vi "PadString.vi"(9 "size":i32=8, 11 "data":string) -> (3 "String":string)   [LabVIEW 2022 SP3]
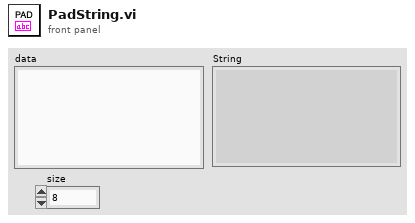
[diagram p1: front panel]
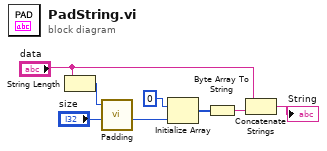
[diagram p0: block diagram]
diagram:
  n1 = String Length(string="data") -> (length=w6:i32)
  n2 = call "Padding.vi"("size"="size", "bytes in"=w6) -> ("padding"=w2:i32)  [unwired: 8 in, 1 out]
  n3 = Initialize Array(u8 0 ("element"), w2) -> (w4:u8[])
  n4 = Byte Array To String(unsigned byte array=w4) -> (string=w7:string)
  n5 = Concatenate Strings("data", w7) -> (→"String":string)
